vi "XY Graph Remove Data Point from Plot.vi"(8 "Error In":errorcluster, 9 "Point":cluster{"X":dbl, "Y":dbl}, 11 "Plot in":cluster{"X Array":dbl[], "Y Array":dbl[]}) -> (0 "Error Out":errorcluster, 1 "Point  Index":i32, 2 "Distance to Plot":dbl, 3 "Plot out":cluster{"X Array":dbl[], "Y Array":dbl[]})   [LabVIEW 2021, in "XY Graph Add-Ons.lvlib"]
uses:
  XY Graph Add-Ons.lvlib
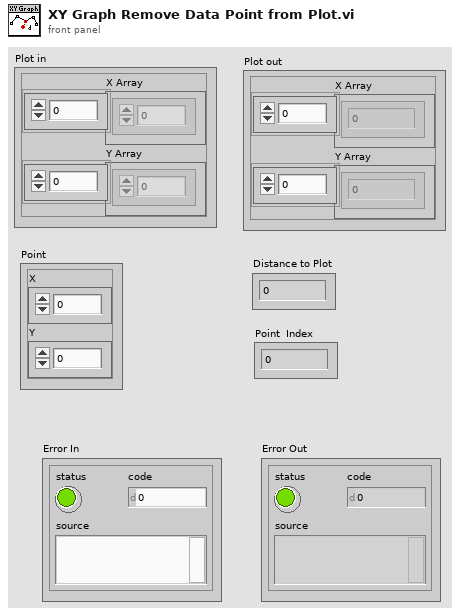
[diagram p1: front panel]
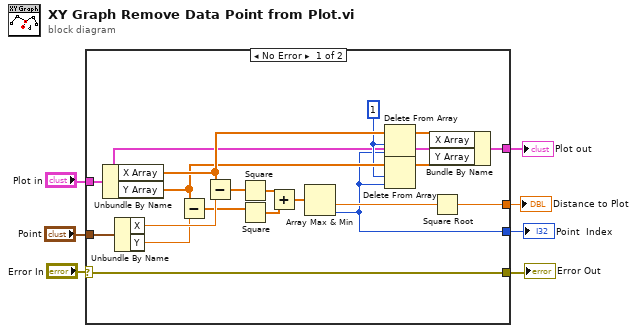
[diagram p0: block diagram]
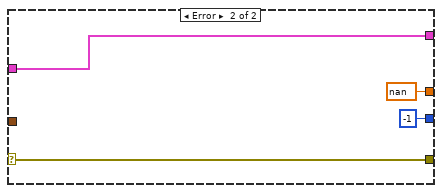
[diagram p2: hidden frame]
diagram:
  n1 = case shown="No Error" "Error In" {
    selector: "Error In" -> [w9 w30]
    tunnel: "Point" -> [w26 _]
    tunnel: [w17 nan] -> w6
    tunnel: "Plot in" -> [w13 w29]
    tunnel: [w10 w29] -> w4
    tunnel: [w9 w30] -> w2
    tunnel: [w8 -1] -> w1
    frame No Error {
      w14 = 1 ("length")
      n2 = Unbundle By Name(w13) -> ("X Array"=w16:dbl[], "Y Array"=w15:dbl[])
      n3 = Unbundle By Name(w26) -> ("X"=w25:dbl, "Y"=w24:dbl)
      n4 = Subtract(x=w15, y=w24) -> (x-y=w22:dbl[])
      n5 = Subtract(x=w16, y=w25) -> (x-y=w23:dbl[])
      n6 = Square(x=w23) -> (x^2=w21:dbl[])
      n7 = Square(x=w22) -> (x^2=w20:dbl[])
      n8 = Add(x=w21, y=w20) -> (x+y=w19:dbl[])
      n9 = Array Max & Min(array=w19) -> (min value=w18:dbl, min index (indices)=w8:i32)  [unwired: 2 out]
      n10 = Delete From Array(array=w16, length=w14, index=w8) -> (array with subset deleted=w12:dbl[])  [unwired: 1 out]
      n11 = Delete From Array(array=w15, length=w14, index=w8) -> (array with subset deleted=w11:dbl[])  [unwired: 1 out]
      n12 = Bundle By Name(cluster=w13, "X Array"=w12, "Y Array"=w11) -> (w10:cluster{"X Array":dbl[], "Y Array":dbl[]})
      n13 = Square Root(x=w18) -> (sqrt(x)=w17:dbl)
    }
    frame Error {
    }
  }
  "Plot out" <- w4
  "Error Out" <- w2
  "Distance to Plot" <- w6
  "Point  Index" <- w1
